vi "PCO_Description3.vi"() -> (0 "PCO_Description3":T2, 1 "PCO_Description3_Raw":T1, 2 "Length":u16, 3 "Raw_Length":u16)   [LabVIEW 2020, in "SDK.lvlib" / "Structures.lvlib"]
doc: "Use this template to build a VI to use as a subVI."
uses:
  Structures.lvlib
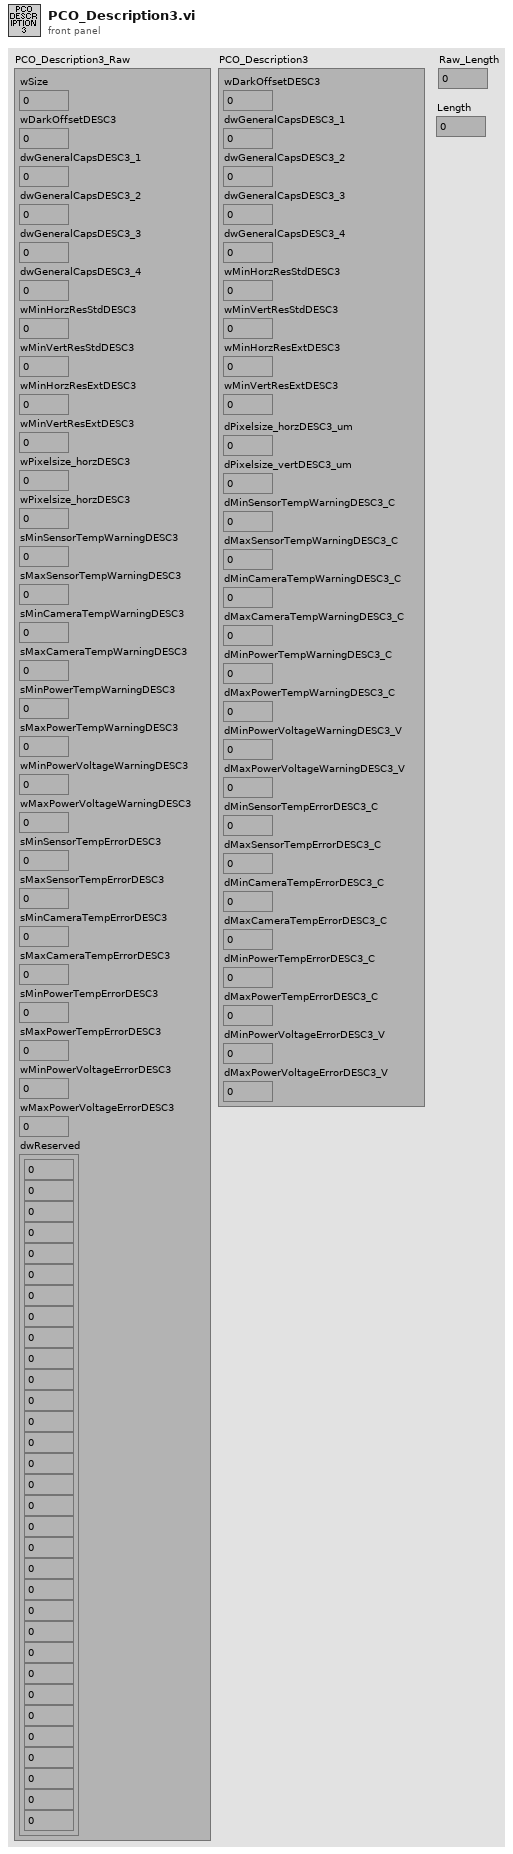
[diagram p1: front panel]
types:
  T1 = cluster{"wSize":u16, "wDarkOffsetDESC3":u16, "dwGeneralCapsDESC3_1":u32, "dwGeneralCapsDESC3_2":u32, "dwGeneralCapsDESC3_3":u32, "dwGeneralCapsDESC3_4":u32, "wMinHorzResStdDESC3":u16, "wMinVertResStdDESC3":u16, "wMinHorzResExtDESC3":u16, "wMinVertResExtDESC3":u16, "wPixelsize_horzDESC3":u16, "wPixelsize_horzDESC3":u16, "sMinSensorTempWarningDESC3":i16, "sMaxSensorTempWarningDESC3":i16, "sMinCameraTempWarningDESC3":i16, "sMaxCameraTempWarningDESC3":i16, "sMinPowerTempWarningDESC3":i16, "sMaxPowerTempWarningDESC3":i16, "wMinPowerVoltageWarningDESC3":u16, "wMaxPowerVoltageWarningDESC3":u16, "sMinSensorTempErrorDESC3":i16, "sMaxSensorTempErrorDESC3":i16, "sMinCameraTempErrorDESC3":i16, "sMaxCameraTempErrorDESC3":i16, "sMinPowerTempErrorDESC3":i16, "sMaxPowerTempErrorDESC3":i16, "wMinPowerVoltageErrorDESC3":u16, "wMaxPowerVoltageErrorDESC3":u16, "dwReserved":cluster{u32, u32, u32, u32, u32, u32, u32, u32, u32, u32, u32, u32, u32, u32, u32, u32, u32, u32, u32, u32, u32, u32, u32, u32, u32, u32, u32, u32, u32, u32, u32, u32}}
  T2 = cluster{"wDarkOffsetDESC3":u16, "dwGeneralCapsDESC3_1":u32, "dwGeneralCapsDESC3_2":u32, "dwGeneralCapsDESC3_3":u32, "dwGeneralCapsDESC3_4":u32, "wMinHorzResStdDESC3":u16, "wMinVertResStdDESC3":u16, "wMinHorzResExtDESC3":u16, "wMinVertResExtDESC3":u16, "dPixelsize_horzDESC3_um":dbl, "dPixelsize_vertDESC3_um":dbl, "dMinSensorTempWarningDESC3_C":dbl, "dMaxSensorTempWarningDESC3_C":dbl, "dMinCameraTempWarningDESC3_C":dbl, "dMaxCameraTempWarningDESC3_C":dbl, "dMinPowerTempWarningDESC3_C":dbl, "dMaxPowerTempWarningDESC3_C":dbl, "dMinPowerVoltageWarningDESC3_V":dbl, "dMaxPowerVoltageWarningDESC3_V":dbl, "dMinSensorTempErrorDESC3_C":dbl, "dMaxSensorTempErrorDESC3_C":dbl, "dMinCameraTempErrorDESC3_C":dbl, "dMaxCameraTempErrorDESC3_C":dbl, "dMinPowerTempErrorDESC3_C":dbl, "dMaxPowerTempErrorDESC3_C":dbl, "dMinPowerVoltageErrorDESC3_V":dbl, "dMaxPowerVoltageErrorDESC3_V":dbl}
  T3 = cluster{u32, u32, u32, u32, u32, u32, u32, u32, u32, u32, u32, u32, u32, u32, u32, u32, u32, u32, u32, u32, u32, u32, u32, u32, u32, u32, u32, u32, u32, u32, u32, u32}
  T4 = cluster{"wDarkOffsetDESC3":u16, "dwGeneralCapsDESC3_1":u32, "dwGeneralCapsDESC3_2":u32, "dwGeneralCapsDESC3_3":u32, "dwGeneralCapsDESC3_4":u32, "wMinHorzResStdDESC3":u16, "wMinVertResStdDESC3":u16, "wMinHorzResExtDESC3":u16, "wMinVertResExtDESC3":u16, dbl, dbl, dbl, dbl, dbl, dbl, dbl, dbl, dbl, dbl, dbl, dbl, dbl, dbl, dbl, dbl, dbl, dbl}
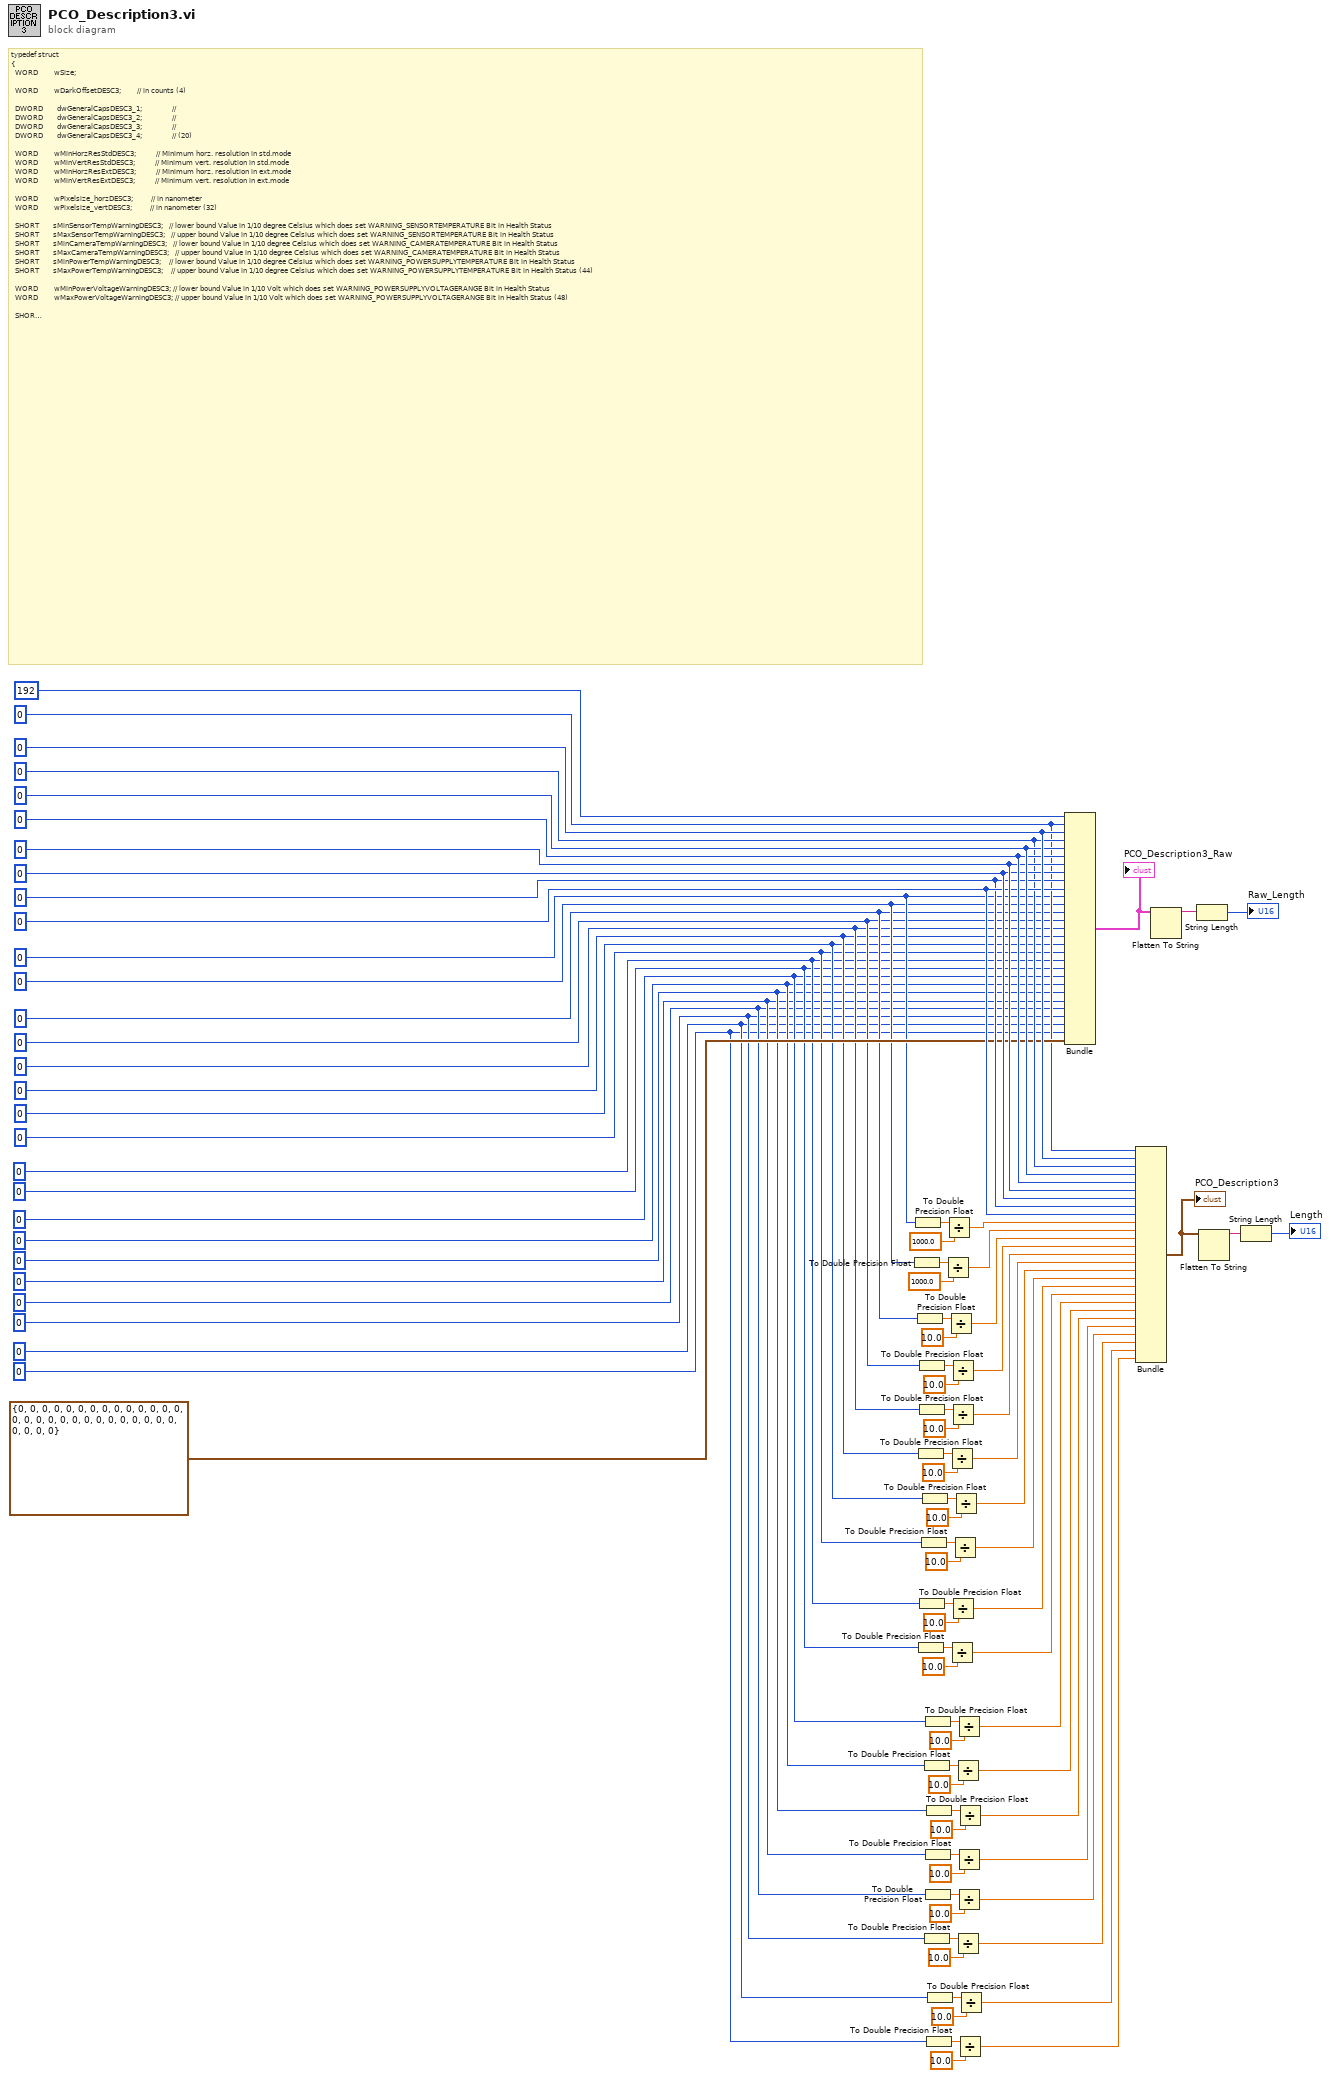
[diagram p0: block diagram]
diagram:
  w11 = u16 0 ("wMaxPowerVoltageErrorDESC3")
  w12 = u16 0 ("wMinPowerVoltageErrorDESC3")
  w13 = i16 0 ("sMaxPowerTempErrorDESC3")
  w14 = i16 0 ("sMinPowerTempErrorDESC3")
  w15 = i16 0 ("sMaxCameraTempErrorDESC3")
  w16 = i16 0 ("sMinCameraTempErrorDESC3")
  w17 = i16 0 ("sMaxSensorTempErrorDESC3")
  w18 = i16 0 ("sMinSensorTempErrorDESC3")
  w19 = u16 0 ("wMaxPowerVoltageWarningDESC3")
  w20 = u16 0 ("wMinPowerVoltageWarningDESC3")
  w47 = i16 0 ("sMaxPowerTempWarningDESC3")
  w48 = i16 0 ("sMinPowerTempWarningDESC3")
  w49 = i16 0 ("sMaxCameraTempWarningDESC3")
  w50 = i16 0 ("sMinCameraTempWarningDESC3")
  w51 = i16 0 ("sMaxSensorTempWarningDESC3")
  w52 = i16 0 ("sMinSensorTempWarningDESC3")
  w66 = u16 0 ("wPixelsize_horzDESC3")
  w72 = u16 0 ("wPixelsize_horzDESC3")
  w78 = u16 0 ("wMinVertResExtDESC3")
  w76 = u16 0 ("wMinHorzResExtDESC3")
  w79 = u16 0 ("wMinVertResStdDESC3")
  w80 = u16 0 ("wMinHorzResStdDESC3")
  w81 = u32 0 ("dwGeneralCapsDESC3_4")
  w82 = u32 0 ("dwGeneralCapsDESC3_3")
  w75 = u32 0 ("dwGeneralCapsDESC3_2")
  w83 = u32 0 ("dwGeneralCapsDESC3_1")
  w73 = u16 0 ("wDarkOffsetDESC3")
  # "typedef struct\n{\n  WORD        wSize;\n\n  WORD        wDarkOffsetDESC3;        // in counts (4)\n\n  DWORD       dwGeneralCapsDESC3_1;               // \n  DWORD       dwGeneralCapsDESC3_2;               // \n  DWORD       dwGeneralCapsDESC3_3;               // \n  DWORD       dwGeneralCapsDESC3_4;               // (20)\n\n  WORD        wMinHorzResStdDESC3;          // Minimum horz. resolution in std.mode\n  WORD        wMinVertResStdDESC3;          // Minimum vert. resolution in std.mode\n  WORD        wMinHorzResExtDESC3;          // Minimum horz. resolution in ext.mode\n  WORD        wMinVertResExtDESC3;          // Minimum vert. resolution in ext.mode\n\n  WORD        wPixelsize_horzDESC3;         // in nanometer\n  WORD        wPixelsize_vertDESC3;         // in nanometer (32)\n\n  SHORT       sMinSensorTempWarningDESC3;   // lower bound Value in 1/10 degree Celsius which does set WARNING_SENSORTEMPERATURE Bit in Health Status\n  SHORT       sMaxSensorTempWarningDESC3;   // upper bound Value in 1/10 degree Celsius which does set WARNING_SENSORTEMPERATURE Bit in Health Status\n  SHORT       sMinCameraTempWarningDESC3;   // lower bound Value in 1/10 degree Celsius which does set WARNING_CAMERATEMPERATURE Bit in Health Status\n  SHORT       sMaxCameraTempWarningDESC3;   // upper bound Value in 1/10 degree Celsius which does set WARNING_CAMERATEMPERATURE Bit in Health Status\n  SHORT       sMinPowerTempWarningDESC3;    // lower bound Value in 1/10 degree Celsius which does set WARNING_POWERSUPPLYTEMPERATURE Bit in Health Status\n  SHORT       sMaxPowerTempWarningDESC3;    // upper bound Value in 1/10 degree Celsius which does set WARNING_POWERSUPPLYTEMPERATURE Bit in Health Status (44)\n\n  WORD        wMinPowerVoltageWarningDESC3; // lower bound Value in 1/10 Volt which does set WARNING_POWERSUPPLYVOLTAGERANGE Bit in Health Status\n  WORD        wMaxPowerVoltageWarningDESC3; // upper bound Value in 1/10 Volt which does set WARNING_POWERSUPPLYVOLTAGERANGE Bit in Health Status (48)\n\n  SHORT       sMinSensorTempErrorDESC3;     // lower bound Value in 1/10 degree Celsius which does set ERROR_SENSORTEMPERATURE Bit in Health Status\n  SHORT       sMaxSensorTempErrorDESC3;     // upper bound Value in 1/10 degree Celsius which does set ERROR_SENSORTEMPERATURE Bit in Health Status\n  SHORT       sMinCameraTempErrorDESC3;     // lower bound Value in 1/10 degree Celsius which does set ERROR_CAMERATEMPERATURE Bit in Health Status\n  SHORT       sMaxCameraTempErrorDESC3;     // upper bound Value in 1/10 degree Celsius which does set ERROR_CAMERATEMPERATURE Bit in Health Status\n  SHORT       sMinPowerTempErrorDESC3;      // lower bound Value in 1/10 degree Celsius which does set ERROR_POWERSUPPLYTEMPERATURE Bit in Health Status\n  SHORT       sMaxPowerTempErrorDESC3;      // upper bound Value in 1/10 degree Celsius which does set ERROR_POWERSUPPLYTEMPERATURE Bit in Health Status (60)\n\n  WORD        wMinPowerVoltageErrorDESC3;   // lower bound Value in 1/10 Volt which does set ERROR_POWERSUPPLYVOLTAGERANGE Bit in Health Status\n  WORD        wMaxPowerVoltageErrorDESC3;   // upper bound Value in 1/10 Volt which does set ERROR_POWERSUPPLYVOLTAGERANGE Bit in Health Status (64)\n\n  DWORD       dwReserved[32];               // (192)\n} PCO_Description3;"
  n1 = To Double Precision Float(number=w66) -> (double precision float=w67:dbl)
  n2 = To Double Precision Float(number=w72) -> (double precision float=w71:dbl)
  n3 = To Double Precision Float(number=w52) -> (double precision float=w63:dbl)
  n4 = To Double Precision Float(number=w49) -> (double precision float=w57:dbl)
  n5 = To Double Precision Float(number=w19) -> (double precision float=w37:dbl)
  n6 = To Double Precision Float(number=w51) -> (double precision float=w61:dbl)
  n7 = To Double Precision Float(number=w50) -> (double precision float=w59:dbl)
  n8 = To Double Precision Float(number=w20) -> (double precision float=w39:dbl)
  n9 = To Double Precision Float(number=w47) -> (double precision float=w53:dbl)
  n10 = To Double Precision Float(number=w48) -> (double precision float=w55:dbl)
  n11 = To Double Precision Float(number=w17) -> (double precision float=w33:dbl)
  n12 = To Double Precision Float(number=w13) -> (double precision float=w25:dbl)
  n13 = To Double Precision Float(number=w18) -> (double precision float=w35:dbl)
  n14 = To Double Precision Float(number=w15) -> (double precision float=w29:dbl)
  n15 = To Double Precision Float(number=w14) -> (double precision float=w27:dbl)
  n16 = To Double Precision Float(number=w16) -> (double precision float=w31:dbl)
  n17 = To Double Precision Float(number=w11) -> (double precision float=w21:dbl)
  n18 = To Double Precision Float(number=w12) -> (double precision float=w23:dbl)
  n19 = Divide(x=w67, y=1000.0) -> (x/y=w65:dbl)
  n20 = Divide(x=w71, y=1000.0) -> (x/y=w69:dbl)
  n21 = Divide(x=w63, y=10.0) -> (x/y=w46:dbl)
  n22 = Divide(x=w57, y=10.0) -> (x/y=w43:dbl)
  n23 = Divide(x=w37, y=10.0) -> (x/y=w9:dbl)
  n24 = Divide(x=w61, y=10.0) -> (x/y=w45:dbl)
  n25 = Divide(x=w59, y=10.0) -> (x/y=w44:dbl)
  n26 = Divide(x=w39, y=10.0) -> (x/y=w10:dbl)
  n27 = Divide(x=w53, y=10.0) -> (x/y=w41:dbl)
  n28 = Divide(x=w55, y=10.0) -> (x/y=w42:dbl)
  n29 = Divide(x=w33, y=10.0) -> (x/y=w7:dbl)
  n30 = Divide(x=w25, y=10.0) -> (x/y=w3:dbl)
  n31 = Divide(x=w35, y=10.0) -> (x/y=w8:dbl)
  n32 = Divide(x=w29, y=10.0) -> (x/y=w5:dbl)
  n33 = Divide(x=w27, y=10.0) -> (x/y=w4:dbl)
  n34 = Divide(x=w31, y=10.0) -> (x/y=w6:dbl)
  n35 = Divide(x=w21, y=10.0) -> (x/y=w1:dbl)
  n36 = Divide(x=w23, y=10.0) -> (x/y=w2:dbl)
  n37 = Bundle("wSize"=u16 192, "wDarkOffsetDESC3"=w73, "dwGeneralCapsDESC3_1"=w83, "dwGeneralCapsDESC3_2"=w75, "dwGeneralCapsDESC3_3"=w82, "dwGeneralCapsDESC3_4"=w81, "wMinHorzResStdDESC3"=w80, "wMinVertResStdDESC3"=w79, "wMinHorzResExtDESC3"=w76, "wMinVertResExtDESC3"=w78, "wPixelsize_horzDESC3"=w72, "wPixelsize_horzDESC3"=w66, "sMinSensorTempWarningDESC3"=w52, "sMaxSensorTempWarningDESC3"=w51, "sMinCameraTempWarningDESC3"=w50, "sMaxCameraTempWarningDESC3"=w49, "sMinPowerTempWarningDESC3"=w48, "sMaxPowerTempWarningDESC3"=w47, "wMinPowerVoltageWarningDESC3"=w20, "wMaxPowerVoltageWarningDESC3"=w19, "sMinSensorTempErrorDESC3"=w18, "sMaxSensorTempErrorDESC3"=w17, "sMinCameraTempErrorDESC3"=w16, "sMaxCameraTempErrorDESC3"=w15, "sMinPowerTempErrorDESC3"=w14, "sMaxPowerTempErrorDESC3"=w13, "wMinPowerVoltageErrorDESC3"=w12, "wMaxPowerVoltageErrorDESC3"=w11, "dwReserved"=T3 {0, 0, 0, 0, 0, 0, 0, 0, 0, 0, 0, 0, 0, 0, 0, 0, 0, 0, 0, 0, 0, 0, 0, 0, 0, 0, 0, 0, 0, 0, 0, 0}) -> (w77:T1)  [unwired: 1 in]
  "PCO_Description3_Raw" <- w77
  n38 = Bundle("wDarkOffsetDESC3"=w73, "dwGeneralCapsDESC3_1"=w83, "dwGeneralCapsDESC3_2"=w75, "dwGeneralCapsDESC3_3"=w82, "dwGeneralCapsDESC3_4"=w81, "wMinHorzResStdDESC3"=w80, "wMinVertResStdDESC3"=w79, "wMinHorzResExtDESC3"=w76, "wMinVertResExtDESC3"=w78, w69, w65, w46, w45, w44, w43, w42, w41, w10, w9, w8, w7, w6, w5, w4, w3, w2, w1) -> (w89:T4)  [unwired: 1 in]
  "PCO_Description3" <- w89
  n39 = Flatten To String(anything=w77) -> (data string=w87:string)  [unwired: 3 in, 2 out]
  n40 = String Length(string=w87) -> (length=→"Raw_Length":i32)
  n41 = Flatten To String(anything=w89) -> (data string=w88:string)  [unwired: 3 in, 2 out]
  n42 = String Length(string=w88) -> (length=→"Length":i32)
